vi "practica3.vi"() -> ()   [LabVIEW 2018]
uses:
  <vilib>/Analysis/Matrix/Datatypes/RealMatrix.ctl
  <vilib>/Utility/file.llb/Read Delimited Spreadsheet (DBL).vi
  <vilib>/Analysis/Matrix/Numeric/Conversions/Array To Matrix - RA2.vi
  <vilib>/Analysis/Matrix/Numeric/Conversions/Matrix To Array - RM.vi
  <vilib>/Utility/file.llb/Write Delimited Spreadsheet (DBL).vi
  <vilib>/Analysis/Matrix/NI_Matrix.lvlib
panel:
  in  "file (use dialog) 2":path
  out "cluster":T1
  out "Real Matrix":T2
  out "subarray":dbl[][](array[numeric])
  out "all rows":dbl[][](array[numeric])
  out "first row":dbl[](array[numeric])
  in  "file (use dialog)":path
  out "text":string
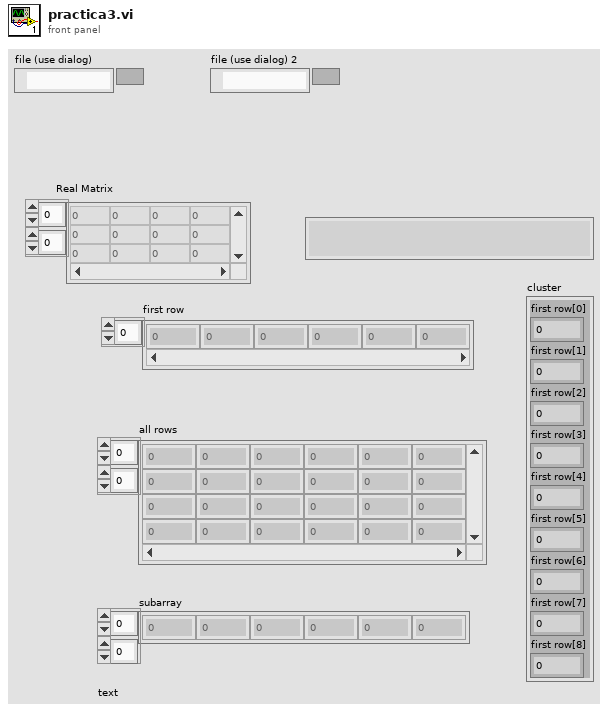
[diagram p1: front panel]
types:
  T1 = cluster{"first row[0]":dbl, "first row[1]":dbl, "first row[2]":dbl, "first row[3]":dbl, "first row[4]":dbl, "first row[5]":dbl, "first row[6]":dbl, "first row[7]":dbl, "first row[8]":dbl}
  T2 = typedef "NI_Matrix.lvlib/RealMatrix.ctl" = dbl[][]
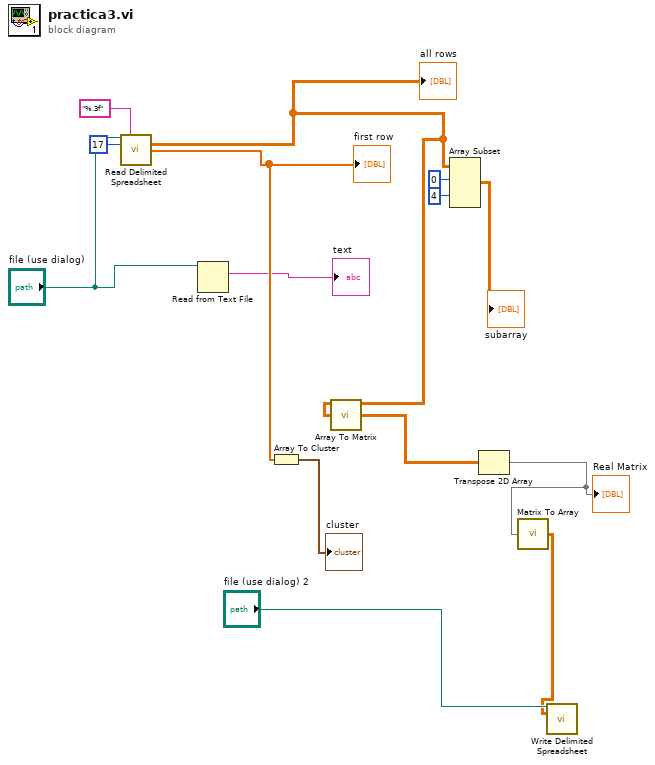
[diagram p0: block diagram]
diagram:
  n1 = call-poly <vilib>:"Read Delimited Spreadsheet.vi"("file path (dialog if empty)"="file (use dialog)", "format (%.3f)"="%.3f", "number of rows (all:-1)"=17) -> ("all rows"=w4:dbl[][], "first row"=w9:dbl[])  [unwired: 7 in, 4 out]
  "first row" <- w9
  "all rows" <- w4
  n2 = Read from Text File(file (use dialog)="file (use dialog)") -> (text=→"text":string)  [unwired: 3 in, 3 out]
  n3 = Array To Cluster(array=w9) -> (cluster=→"cluster":T1)
  n4 = call-poly <vilib>:"Array To Matrix.vi"("Real 2D Array"=w4) -> ("Real Matrix"=w2:T2)
  n5 = Array Subset(array=w4, index (row)=0 ("index"), index (col)=4 ("index")) -> (→"subarray":dbl[][])  [unwired: 2 in]
  n6 = Transpose 2D Array(2D array=w2) -> (transposed array=w1:T2)
  "Real Matrix" <- w1
  n7 = call-poly <vilib>:"Matrix To Array.vi"("Real Matrix"=w1) -> ("Real 2D Array"=w5:dbl[][])
  n8 = call-poly <vilib>:"Write Delimited Spreadsheet.vi"("file path (dialog if empty)"="file (use dialog) 2", "2D data"=w5) -> ()  [unwired: 12 in, 2 out]
